vi "Write Channels_ AO.vi"(8 "error in (no error)":errorcluster, 10 "Channels: AO":T1 {"Phase" format="%.3g"; "Frequency" min=0.0001 max=10000.0 format="%.3g"; "Offset" format="%.3p"; "Amplitude" min=0.0 max=10.0 format="%.3p"}, 11 "Lockin.DAQ":refnum<class "Lockin.DAQ.lvclass">) -> (0 "error out":errorcluster, 3 "Lockin.DAQ out":refnum<class "Lockin.DAQ.lvclass">)   [LabVIEW 2016, in "Lockin.DAQ.lvclass"]
uses:
  Lockin.DAQ.lvclass
  Typedefs/AO-cluster.ctl
  Instrument.Lockinl.UI/Typedefs/AO Channel--Cluster.ctl
  Typedefs/Function-enum.ctl
  Lockin.DAQ.lvclass/Lockin.DAQ.ctl
  Instrument.Lockinl.UI/Instrument.Lockin.UI.lvclass
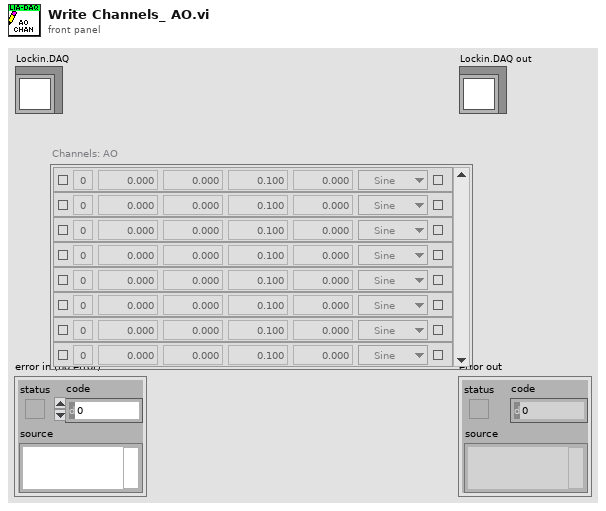
[diagram p1: front panel]
types:
  T1 = typedef "Lockin.DAQ.lvclass/AO-cluster.ctl" = T2[]
  T2 = typedef "Instrument.Lockin.UI.lvclass/AO Channel--Cluster.ctl" = cluster{"Enable?":bool, "Channel":i32, "Amplitude":dbl, "Offset":dbl, "Frequency":dbl, "Phase":dbl, "Function":T3, "Sweeping?":bool}
  T3 = typedef "Lockin.DAQ.lvclass/Function-enum.ctl" = enum16{"Sine", "Triangle", "Square"}
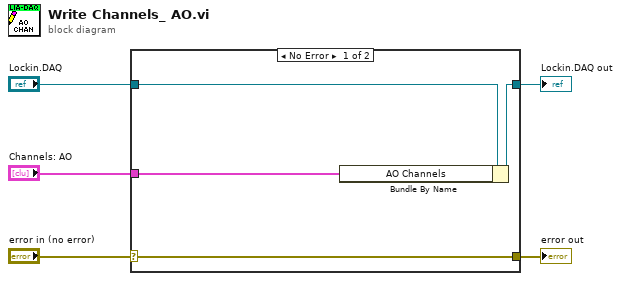
[diagram p0: block diagram]
diagram:
  n1 = case shown="No Error" "error in (no error)" {
    selector: "error in (no error)" -> [w9 w10]
    tunnel: [w9 w10] -> w4
    tunnel: [w7 w11] -> w2
    tunnel: "Lockin.DAQ" -> [w8 w11]
    tunnel: "Channels: AO" -> [w6 _]
    frame No Error {
      n2 = Bundle By Name(cluster=w8, "AO Channels"=w6) -> (w7:refnum<class "Lockin.DAQ.lvclass">)
    }
    frame Error {
    }
  }
  "error out" <- w4
  "Lockin.DAQ out" <- w2
